vi "Teleop.vi"(10 "Match Info":T1={"Autonomous Elapsed Seconds"=0.0, "TeleOp Elapsed Seconds"=0.0, "Disabled Elapsed Seconds"=0.0, "Visited Autonomous"=FALSE, "Visited TeleOp"=FALSE, "Visited Disabled"=FALSE, "Autonomous Settings"={"Autonomous Style"=enum."Independent", "VI Refnum"=refnum}}, 11 "Call Context":T2) -> ()   [LabVIEW 2013]
doc: "This VI is called for each TeleOp packet received from the DS where the robot is not disabled. It is often used to read from the joysticks and update I/O or to update setpoints for timed control loops. It should complete and return within 20 milliseconds or it may miss DS packets."
uses:
  <vilib>/Rock Robotics/WPI/DriverStation/WPI_DriverStationDerivedRobotMode.ctl
  <vilib>/Rock Robotics/WPI/DriverStation/WPI_DriverStationMatch Info.ctl
  <vilib>/Rock Robotics/WPI/Solenoid/WPI_SolenoidValue.ctl
  Robot Global Data.vi
  <vilib>/Rock Robotics/WPI/Solenoid/WPI_SolenoidSetEnum.vi
  <vilib>/Rock Robotics/WPI/Joystick/WPI_JoystickGetSetRefNum.vi
  <vilib>/Rock Robotics/WPI/RobotDrive/WPI_RobotDriveArcadeDrive_Standard(NoSaturation).vi
  <vilib>/Rock Robotics/WPI/RobotDrive/WPI_RobotDriveGetSetRefNum.vi
panel:
  out "Piston 2":bool
  out "Piston 3":bool
  out "Piston 1":bool
  in  "Pneumatics 3":bool
  in  "Pneumatics 2":bool
  in  "Pneumatics 1":bool
  out "axis 2 (y)":dbl
  out "axis 6":dbl
  out "axis 5":dbl
  out "axis 4":dbl
  out "axis 3 (throttle)":dbl
  out "axis 1 (x)":dbl
  out "Numeric 1":dbl(slide) scale=0.0..100.0
  out "Boolean 2":bool
  out "Boolean 1":bool
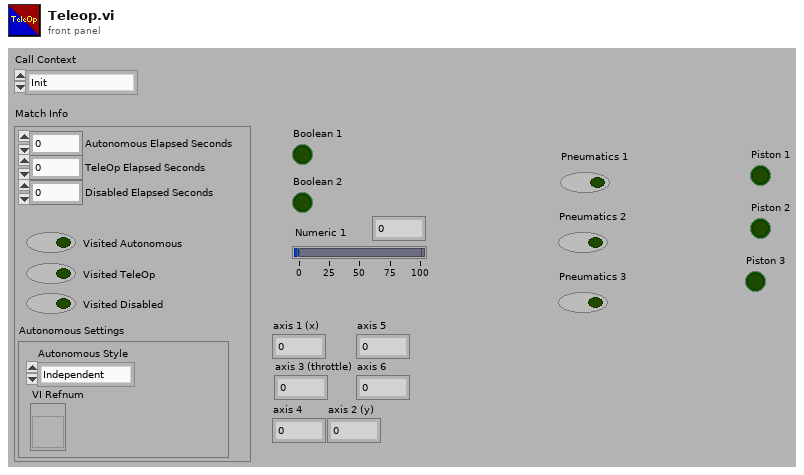
[diagram p1: front panel]
types:
  T1 = typedef "WPI_DriverStationMatch Info.ctl" = cluster{"Autonomous Elapsed Seconds":dbl, "TeleOp Elapsed Seconds":dbl, "Disabled Elapsed Seconds":dbl, "Visited Autonomous":bool, "Visited TeleOp":bool, "Visited Disabled":bool, "Autonomous Settings":cluster{"Autonomous Style":enum16{"Iterative", "Independent"}, "VI Refnum":refnum<vi>}}
  T2 = typedef "WPI_DriverStationDerivedRobotMode.ctl" = enum16{"Init", "Execute", "Stop"}
  T3 = typedef "WPI_SolenoidValue.ctl" = enum16{"Off", "On", "Forward", "Reverse"}
  T4 = typedef "WPI_JoystickDevRef.ctl" = cluster{"Device":T5}
  T5 = typedef "WPI_JoystickDeviceEnum.ctl" = enum16{"USB 1", "USB 2", "USB 3", "USB 4", "Kinect 1", "Kinect 2"}
  T6 = typedef "WPI_JoystickButtonState.ctl" = cluster{"Button 1":bool, "Button 2":bool, "Button 3":bool, "Button 4":bool, "Button 5":bool, "Button 6":bool, "Button 7":bool, "Button 8":bool, "Button 9":bool, "Button 10":bool, "Button 11":bool, "Button 12":bool}
  T7 = cluster{"axis 1 (x)":dbl, "axis 2 (y)":dbl, "axis 3 (throttle)":dbl, "axis 4":dbl, "axis 5":dbl, "axis 6":dbl}
  T8 = typedef "WPI_RobotDriveDevRef.ctl" = cluster{"DevStatus":errorcluster, "Motors[]":T9[], "Square Inputs":bool, "Max Output":dbl, "Isochronous":bool}
  T9 = typedef "WPI_MotorControlDeviceRef.ctl" = cluster{"DeviceStatus":errorcluster, "Type":enum16{"PWM", "CAN"}, "PWM":cluster{"Digital Module":T10, "PWM Channel":T11, "DeadBand":T12}, "CAN":cluster{"Device Number":u8, "Control Mode":T13, "Semaphore":T14, "Max Vout":dbl}, "Invert":bool, "TransformRef":T15, "InvTransformRef":T15}
  T10 = typedef "FPGA_TypedefDigitalModule.ctl" = enum16{"Digital Module 1", "Digital Module 2"}
  T11 = typedef "FPGA_DIOPWMChannel.ctl" = enum8{"PWM 1", "PWM 2", "PWM 3", "PWM 4", "PWM 5", "PWM 6", "PWM 7", "PWM 8", "PWM 9", "PWM 10", "Invalid"}
  T12 = typedef "WPI_PWMDeadband.ctl" = cluster{"Name":string, "maxPositivePwm":i32, "minPositivePwm":i32, "centerPwm":i32, "maxNegativePwm":i32, "minNegativePwm":i32, "angularRange":u16}
  T13 = typedef "WPI_CANJaguar_ControlMode.ctl" = enum8{"Percent VBus", "Current", "Speed", "Position", "Voltage"}
  T14 = typedef "Semaphore RefNum" = refnum<k1>
  T15 = typedef "WPI_PWMTransform_ConPane.ctl" = refnum<vi>
  T16 = typedef "WPI_SolenoidDevRef.ctl" = cluster{"DevStatus":errorcluster, "Solenoid Module":T17, "Forward Solenoid Channel":T18, "Reverse Solenoid Channel":T18}
  T17 = typedef "FPGA_TypedefSolenoidModule.ctl" = enum16{"Solenoid Module 1", "Solenoid Module 2"}
  T18 = typedef "WPI_SolenoidChannel.ctl" = enum8{"Solenoid 1", "Solenoid 2", "Solenoid 3", "Solenoid 4", "Solenoid 5", "Solenoid 6", "Solenoid 7", "Solenoid 8", "Invalid"}
  T19 = typedef "WPI_DigitalInputDevRef.ctl" = cluster{"DevStatus":errorcluster, "DIO Channel":T20, "Digital Module":T10}
  T20 = typedef "FPGA_DIOChannel.ctl" = enum8{"DIO 1", "DIO 2", "DIO 3", "DIO 4", "DIO 5", "DIO 6", "DIO 7", "DIO 8", "DIO 9", "DIO 10", "DIO 11", "DIO 12", "DIO 13", "DIO 14", "Invalid"}
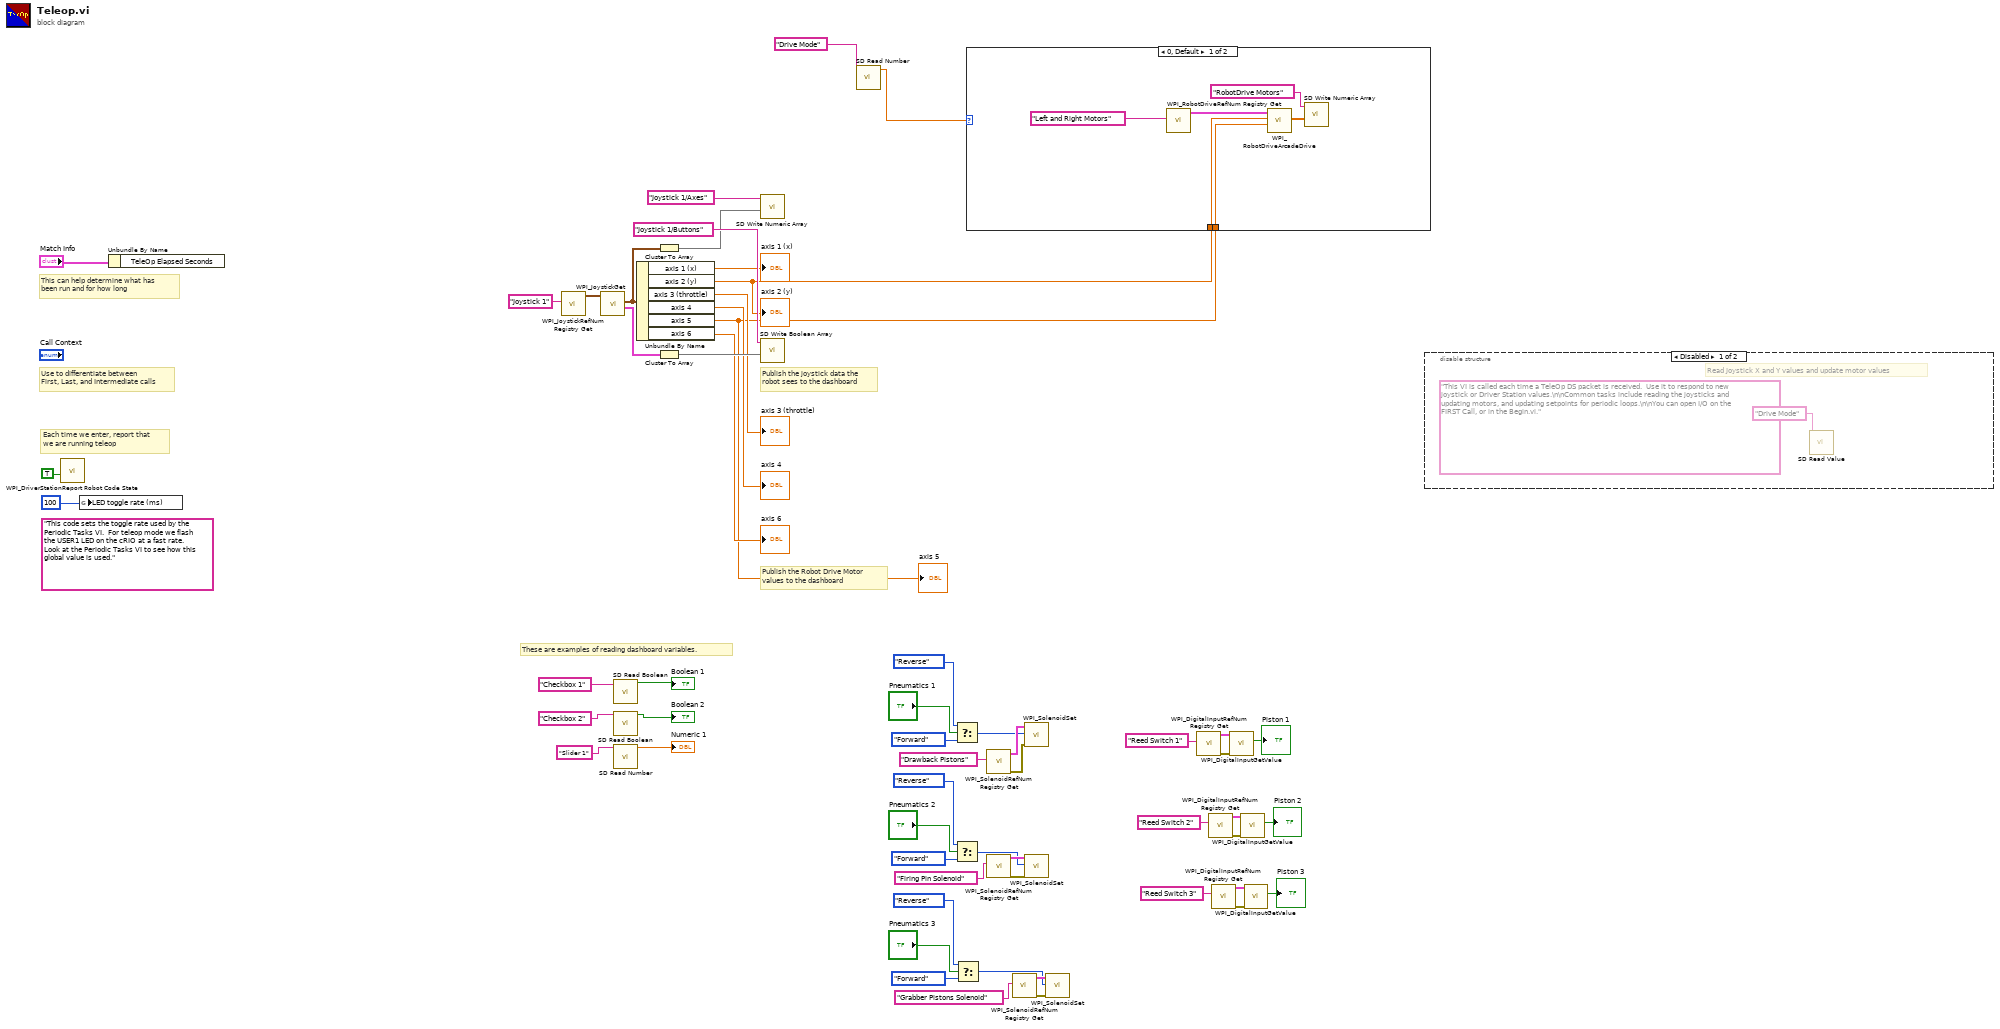
[diagram p0: block diagram]
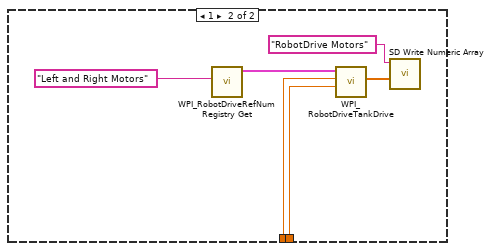
[diagram p2: hidden frame]
diagram:
  (unwired) "This code sets the toggle rate used by the Periodic Tasks VI.  For teleop mode we flash the USER1 LED on the cRIO at a fast rate.  Look at the Periodic Tasks VI to see how this global value is used."
  # "These are examples of reading dashboard variables."
  # "Publish the Robot Drive Motor\nvalues to the dashboard"
  # "Publish the joystick data the\nrobot sees to the dashboard"
  # "Each time we enter, report that\nwe are running teleop"
  # "Use to differentiate between\nFirst, Last, and Intermediate calls"
  # "This can help determine what has\nbeen run and for how long"
  n1 = call <vilib>:"WPI_DriverStationReport Robot Code State.vi"("TeleOp"=TRUE ("Autonomous")) -> ()  [unwired: 10 in, 1 out]
  n2 = global write "Robot Global Data.vi" "LED toggle rate (ms)"(u32 100 ("LED ms toggle rate")) -> ()
  n3 = Unbundle By Name("Match Info") -> ()  [unwired: 1 out]
  n4 = call <vilib>:"WPI_JoystickRefNum Registry Get.vi"("refnum name"="Joystick 1") -> ("JoystickDevRef"=w56:T4)  [unwired: 1 in, 9 out]
  n5 = call <vilib>:"WPI_JoystickGet.vi"("JoystickDevRef"=w56) -> ("Buttons"=w53:T6, "Axes"=w50:T7)  [unwired: 1 in, 4 out]
  n6 = call <vilib>:"SD Read Boolean.vi"("Name"="Checkbox 1" ("refnum name")) -> ("Boolean"=→"Boolean 1":bool)  [unwired: 8 in, 2 out]
  n7 = call <vilib>:"SD Read Boolean.vi"("Name"="Checkbox 2" ("refnum name")) -> ("Boolean"=→"Boolean 2":bool)  [unwired: 8 in, 2 out]
  n8 = call <vilib>:"SD Read Number.vi"("Name"="Slider 1" ("refnum name")) -> ("Numeric"=→"Numeric 1":dbl)  [unwired: 8 in, 2 out]
  n9 = Unbundle By Name(w50) -> ("axis 1 (x)"=→"axis 1 (x)":dbl, "axis 2 (y)"=w41:dbl, "axis 3 (throttle)"=→"axis 3 (throttle)":dbl, "axis 4"=→"axis 4":dbl, "axis 5"=w36:dbl, "axis 6"=→"axis 6":dbl)
  "axis 5" <- w36
  "axis 2 (y)" <- w41
  n10 = Cluster To Array(cluster=w50) -> (array=w49:dbl[])
  n11 = Cluster To Array(cluster=w53) -> (array=w52:bool[])
  n12 = call <vilib>:"SD Write Numeric Array.vi"("Numeric Array"=w49, "Name"="Joystick 1/Axes") -> ()  [unwired: 8 in, 2 out]
  n13 = call <vilib>:"SD Write Boolean Array.vi"("Boolean Array"=w52, "Name"="Joystick 1/Buttons") -> ()  [unwired: 8 in, 2 out]
  n14 = call <vilib>:"SD Read Number.vi"("Name"="Drive Mode") -> ("Numeric"=w35:dbl)  [unwired: 8 in, 2 out]
  n15 = Select(t=WPI_SolenoidValue."Reverse" ("Value"), s="Pneumatics 1", f=WPI_SolenoidValue."Forward") -> (s? t:f=w27:T3)
  n16 = Select(t=WPI_SolenoidValue."Reverse" ("Value"), s="Pneumatics 2", f=WPI_SolenoidValue."Forward") -> (s? t:f=w21:T3)
  n17 = Select(t=WPI_SolenoidValue."Reverse" ("Value"), s="Pneumatics 3", f=WPI_SolenoidValue."Forward") -> (s? t:f=w14:T3)
  n18 = case shown="0, Default" w35 {
    tunnel: w41 -> [w61 w66]
    tunnel: w36 -> [w60 w65]
    frame 0, Default {
      n19 = call <vilib>:"WPI_RobotDriveRefNum Registry Get.vi"("refnum name"="Left and Right Motors") -> ("RobotDriveDevRef"=w62:T8)  [unwired: 1 in, 9 out]
      n20 = call-poly <vilib>:"WPI_RobotDriveArcadeDrive.vi"("Y axis value"=w60, "X axis value"=w61, "RobotDriveDevRef"=w62) -> ("Motor Values"=w59:dbl[])  [unwired: 6 in, 2 out]
      n21 = call <vilib>:"SD Write Numeric Array.vi"("Numeric Array"=w59, "Name"="RobotDrive Motors") -> ()  [unwired: 8 in, 2 out]
    }
    frame 1 {
      n22 = call <vilib>:"WPI_RobotDriveRefNum Registry Get.vi"("refnum name"="Left and Right Motors") -> ("RobotDriveDevRef"=w69:T8)  [unwired: 1 in, 9 out]
      n23 = call <vilib>:"WPI_RobotDriveTankDrive.vi"("Right axis value"=w65, "Left axis value"=w66, "RobotDriveDevRef"=w69) -> ("Motor Values"=w67:dbl[])  [unwired: 6 in, 2 out]
      n24 = call <vilib>:"SD Write Numeric Array.vi"("Numeric Array"=w67, "Name"="RobotDrive Motors") -> ()  [unwired: 8 in, 2 out]
    }
  }
  n25 = call <vilib>:"WPI_SolenoidRefNum Registry Get.vi"("refnum name"="Drawback Pistons") -> ("error out"=w32:errorcluster, "SolenoidDevRef"=w31:T16)  [unwired: 9 in]
  n26 = call <vilib>:"WPI_SolenoidRefNum Registry Get.vi"("refnum name"="Firing Pin Solenoid") -> ("error out"=w26:errorcluster, "SolenoidDevRef"=w25:T16)  [unwired: 9 in]
  n27 = call <vilib>:"WPI_SolenoidRefNum Registry Get.vi"("refnum name"="Grabber Pistons Solenoid") -> ("error out"=w19:errorcluster, "SolenoidDevRef"=w18:T16)  [unwired: 9 in]
  n28 = call-poly <vilib>:"WPI_SolenoidSet.vi"("error in (no error)"=w32, "Value"=w27, "SolenoidDevRef"=w31) -> ()  [unwired: 7 in, 2 out]
  n29 = call-poly <vilib>:"WPI_SolenoidSet.vi"("error in (no error)"=w26, "Value"=w21, "SolenoidDevRef"=w25) -> ()  [unwired: 7 in, 2 out]
  n30 = call-poly <vilib>:"WPI_SolenoidSet.vi"("error in (no error)"=w19, "Value"=w14, "SolenoidDevRef"=w18) -> ()  [unwired: 7 in, 2 out]
  n31 = call <vilib>:"WPI_DigitalInputRefNum Registry Get.vi"("refnum name"="Reed Switch 1") -> ("error out"=w12:errorcluster, "DigitalInputDevRef"=w11:T19)  [unwired: 9 in]
  n32 = call <vilib>:"WPI_DigitalInputRefNum Registry Get.vi"("refnum name"="Reed Switch 2") -> ("error out"=w8:errorcluster, "DigitalInputDevRef"=w7:T19)  [unwired: 9 in]
  n33 = call <vilib>:"WPI_DigitalInputRefNum Registry Get.vi"("refnum name"="Reed Switch 3") -> ("error out"=w4:errorcluster, "DigitalInputDevRef"=w3:T19)  [unwired: 9 in]
  n34 = call <vilib>:"WPI_DigitalInputGetValue.vi"("error in (no error)"=w12, "DigitalInputDevRef"=w11) -> ("Value"=→"Piston 1":bool)  [unwired: 7 in, 2 out]
  n35 = call <vilib>:"WPI_DigitalInputGetValue.vi"("error in (no error)"=w8, "DigitalInputDevRef"=w7) -> ("Value"=→"Piston 2":bool)  [unwired: 7 in, 2 out]
  n36 = call <vilib>:"WPI_DigitalInputGetValue.vi"("error in (no error)"=w4, "DigitalInputDevRef"=w3) -> ("Value"=→"Piston 3":bool)  [unwired: 7 in, 2 out]
  n37 = disable-structure shown="Disabled" {
    frame Disabled {
      (unwired) "This VI is called each time a TeleOp DS packet is received.  Use it to respond to new joystick or Driver Station values.\n\nCommon tasks include reading the joysticks and updating motors, and updating setpoints for periodic loops.\n\nYou can open I/O on the FIRST Call, or in the Begin.vi."
      # "Read Joystick X and Y values and update motor values"
      n38 = call-poly <vilib>:"SD Read Value.vi"("Name"="Drive Mode") -> ("Numeric"=w71:dbl)  [unwired: 8 in, 2 out]
    }
    frame Enabled {
    }
  }
